vi "Read Boolean.vi"(8 "error in":errorcluster, 10 "register name":string, 11 "session in":u32) -> (0 "error out":errorcluster, 2 "value out":bool, 3 "session out":u32)   [LabVIEW 2018, in "Scalar IO Operations.lvlib"]
uses:
  Scalar IO Operations.lvlib
  NiFpga.dll
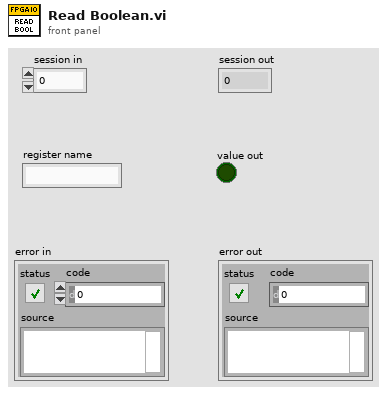
[diagram p1: front panel]
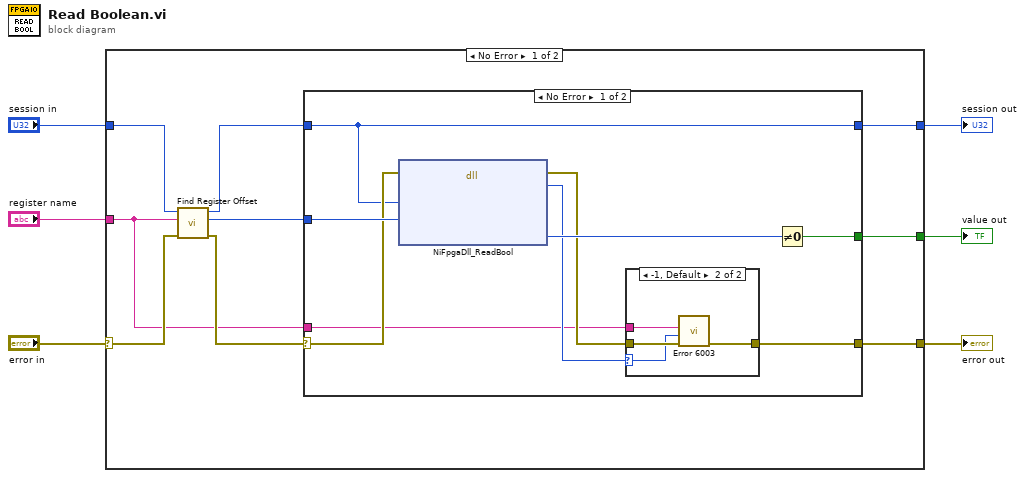
[diagram p0: block diagram]
diagram:
  n1 = case shown="No Error" "error in" {
    selector: "error in" -> [w8 w33]
    tunnel: [w15 w33] -> w6
    tunnel: [w14 w32] -> w5
    tunnel: [w13 _] -> w4
    tunnel: "register name" -> [w7 _]
    tunnel: "session in" -> [w10 w32]
    frame No Error {
      n2 = call "Find Register Offset.vi"("error in (no error)"=w8, "register name"=w7, "session in"=w10) -> ("error out"=w11:errorcluster, "resource offset"=w12:u32, "session out"=w9:u32)  [unwired: 6 in]
      n3 = case shown="No Error" w11 {
        selector: w11 -> [w23 w31]
        tunnel: w9 -> [w22 w30]
        tunnel: [w17 w31] -> w15
        tunnel: [w21 _] -> w13
        tunnel: w12 -> [w24 _]
        tunnel: [w22 w30] -> w14
        tunnel: w7 -> [w16 _]
        frame No Error {
          n4 = dll-call lib="NiFpga.*" fn="NiFpgaDll_ReadBool"(error in=w23, "session"=w22, "offset"=w24) -> (error out=w18:errorcluster, "status"=w19:i32, "value"=w20:u8)  [unwired: 5 in, 1 out]
          n5 = case shown="-1, Default" w19 {
            selector: w19 -> [_ w26]
            tunnel: w18 -> [w25 w29]
            tunnel: [w25 w28] -> w17
            tunnel: w16 -> [_ w27]
            frame 0 {
            }
            frame -1, Default {
              n6 = call "Error 6003.vi"("error in (no error)"=w29, "rio status code"=w26, "register name"=w27) -> ("error out"=w28:errorcluster)  [unwired: 8 in]
            }
          }
          n7 = Not Equal To 0?(x=w20) -> (x != 0?=w21:bool)
        }
        frame Error {
        }
      }
    }
    frame Error {
    }
  }
  "error out" <- w6
  "session out" <- w5
  "value out" <- w4
